vi "uStringManipulation_DO.vi"(8 "error in (no error)":errorcluster, 10 "String in":string, 11 "in":refnum<class "removePrefix.lvclass">) -> (0 "error out":errorcluster, 2 "String":string, 3 "out":refnum<class "removePrefix.lvclass">)   [LabVIEW 2023, in "uStringManipulation_Pack_Std.lvlib" / "removePrefix.lvclass"]
uses:
  removePrefix.lvclass
  removePrefix.lvclass/removePrefix.ctl
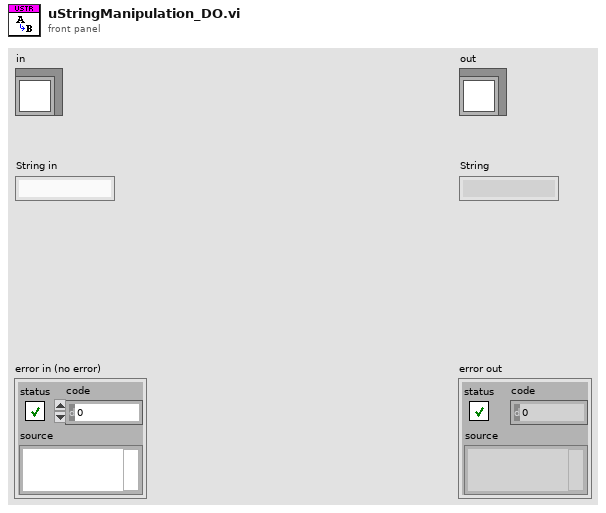
[diagram p1: front panel]
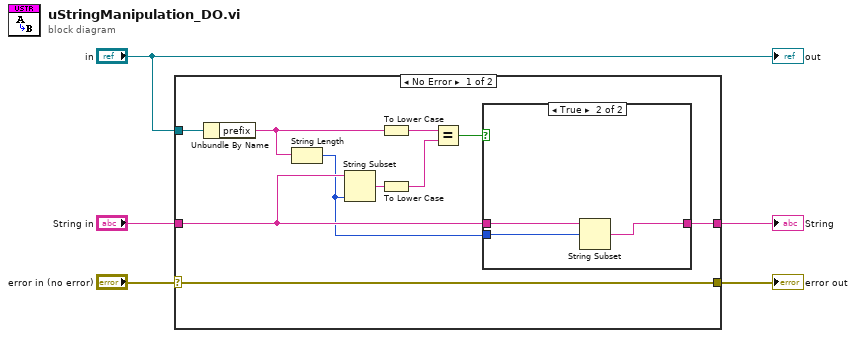
[diagram p0: block diagram]
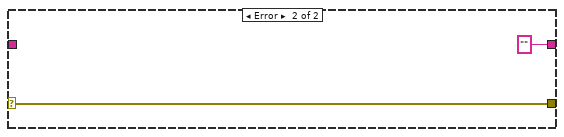
[diagram p3: hidden frame]
diagram:
  n1 = case shown="No Error" "error in (no error)" {
    selector: "error in (no error)" -> [w10 w20]
    tunnel: "String in" -> [w8 _]
    tunnel: [w7 ""] -> w3
    tunnel: "in" -> [w15 _]
    tunnel: [w10 w20] -> w1
    frame No Error {
      n2 = Unbundle By Name(w15) -> ("prefix"=w14:string)
      n3 = String Length(string=w14) -> (length=w6:i32)
      n4 = String Subset(string=w8, length (rest)=w6) -> (substring=w12:string)  [unwired: 1 in]
      n5 = To Lower Case(string=w14) -> (all lower case string=w13:string)
      n6 = To Lower Case(string=w12) -> (all lower case string=w11:string)
      n7 = Equal?(x=w13, y=w11) -> (x = y?=w9:bool)
      n8 = case shown="True" w9 {
        tunnel: w8 -> [w16 w19]
        tunnel: [w16 w18] -> w7
        tunnel: w6 -> [_ w17]
        frame False {
        }
        frame True {
          n9 = String Subset(string=w19, offset (0)=w17) -> (substring=w18:string)  [unwired: 1 in]
        }
      }
    }
    frame Error {
    }
  }
  "error out" <- w1
  "String" <- w3
  "out" <- "in"
